vi "LABVIEW_3VariablesInput.vi"() -> ()   [LabVIEW 2019]
uses:
  <vilib>/Instr/_visa.llb/VISA Configure Serial Port (Instr).vi
panel:
  out "output 3":i32
  out "output 2":i32
  out "output 1":i32
  in  "stop":bool
  out "read buffer":string
  in  "parity (0:none)":enum16{"None", "Odd", "Even", "Mark", "Space"}(ring)
  in  "data bits (8)":u16=8 min=5 max=8 step=1
  in  "baud rate (9600)":u32=9600
  in  "VISA resource name":refnum<visa-resource-name>
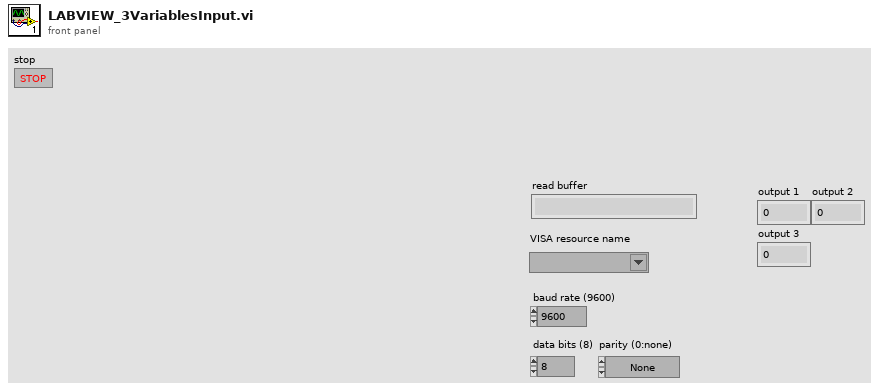
[diagram p1: front panel]
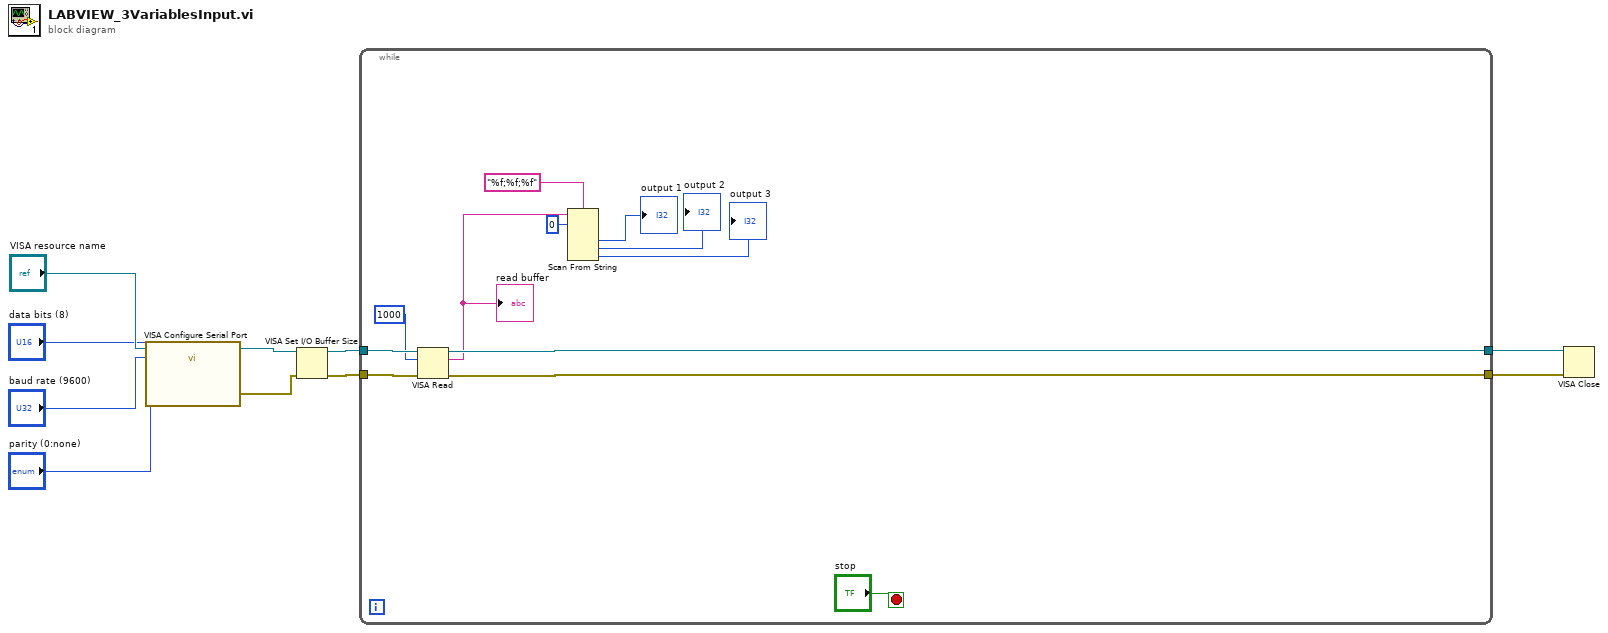
[diagram p0: block diagram]
diagram:
  n1 = call-poly "VISA Configure Serial Port"("VISA resource name"="VISA resource name", "baud rate (9600)"="baud rate (9600)", "data bits (8)"="data bits (8)", "parity (0:none)"="parity (0:none)") -> ("VISA resource name out"=w6:refnum<visa-resource-name>, "error out"=w5:errorcluster)  [unwired: 10 in]
  n2 = VISA Set I/O Buffer Size(VISA resource name=w6, error in (no error)=w5) -> (VISA resource name out=w3:refnum<visa-resource-name>, error out=w4:errorcluster)  [unwired: 2 in]
  n3 = while {
    tunnel: w4 -> [w22]
    tunnel: w3 -> [w21]
    tunnel: [w20] -> w2
    tunnel: [w19] -> w1
    stop <- "stop" stop-if-true
    n4 = VISA Read(VISA resource name=w21, byte count=u32 1000, error in (no error)=w22) -> (VISA resource name out=w20:refnum<visa-resource-name>, read buffer=w16:string, error out=w19:errorcluster)  [unwired: 1 out]
    "read buffer" <- w16
    n5 = Scan From String(format string="%f;%f;%f", input string=w16, initial scan location=u32 0) -> (output 1=→"output 1":i32, output 2=→"output 2":i32, output 3=→"output 3":i32)  [unwired: 4 in, 3 out]
  }
  n6 = VISA Close(VISA resource name=w2, error in (no error)=w1) -> ()  [unwired: 1 out]
